vi "OVEN_Value_Indicator_Update.vi"(6 "Product Code":cluster{string, "ACTUAL  PLC COUNT":i32}[](array[cluster]), 7 "Cluster":T1={"Product List"=[], "SQL reference"=refnum, "Indicator refrence"=[], "Station Number"=[], "Shift Time stamp"=[timestamp(3597615000 s since 1904-01-01), timestamp(3597658199 s since 1904-01-01), timestamp(3597658200 s since 1904-01-01), timestamp(3597614999 s since 1904-01-01), timestamp(3597589800 s since 1904-01-01), timestamp(3597589800 s since 1904-01-01)], "Com Status Station"=[], "ALARAM INDICATOR REF"=[], "Reading"=[], "Read Parameteres"=[], "Station Name"=[], "Oven Read Parameteres"=[]} {"Shift Time stamp" format="%<%X>T"}, 8 "Machine_Number":string, 9 "Numeric":i32, 10 "Array":string[](array[string]), 11 "Cluster in":refnum<vi>) -> (3 "Boolen value of oven":bool)   [LabVIEW 2017]
uses:
  Controls/station_wise_loop_data.ctl
  <vilib>/addons/database/Connection.llb/Conn ObjectReference.ctl
  <vilib>/addons/database/NI_Database_API.lvlib
panel:
  out "400T-2 OVEN COM 2":bool
  out "Machine para Indicator":bool
  in  "Top_zone_1":dbl format="%#_13g"
  out "Read Parameteres 3":string[][](array[string])
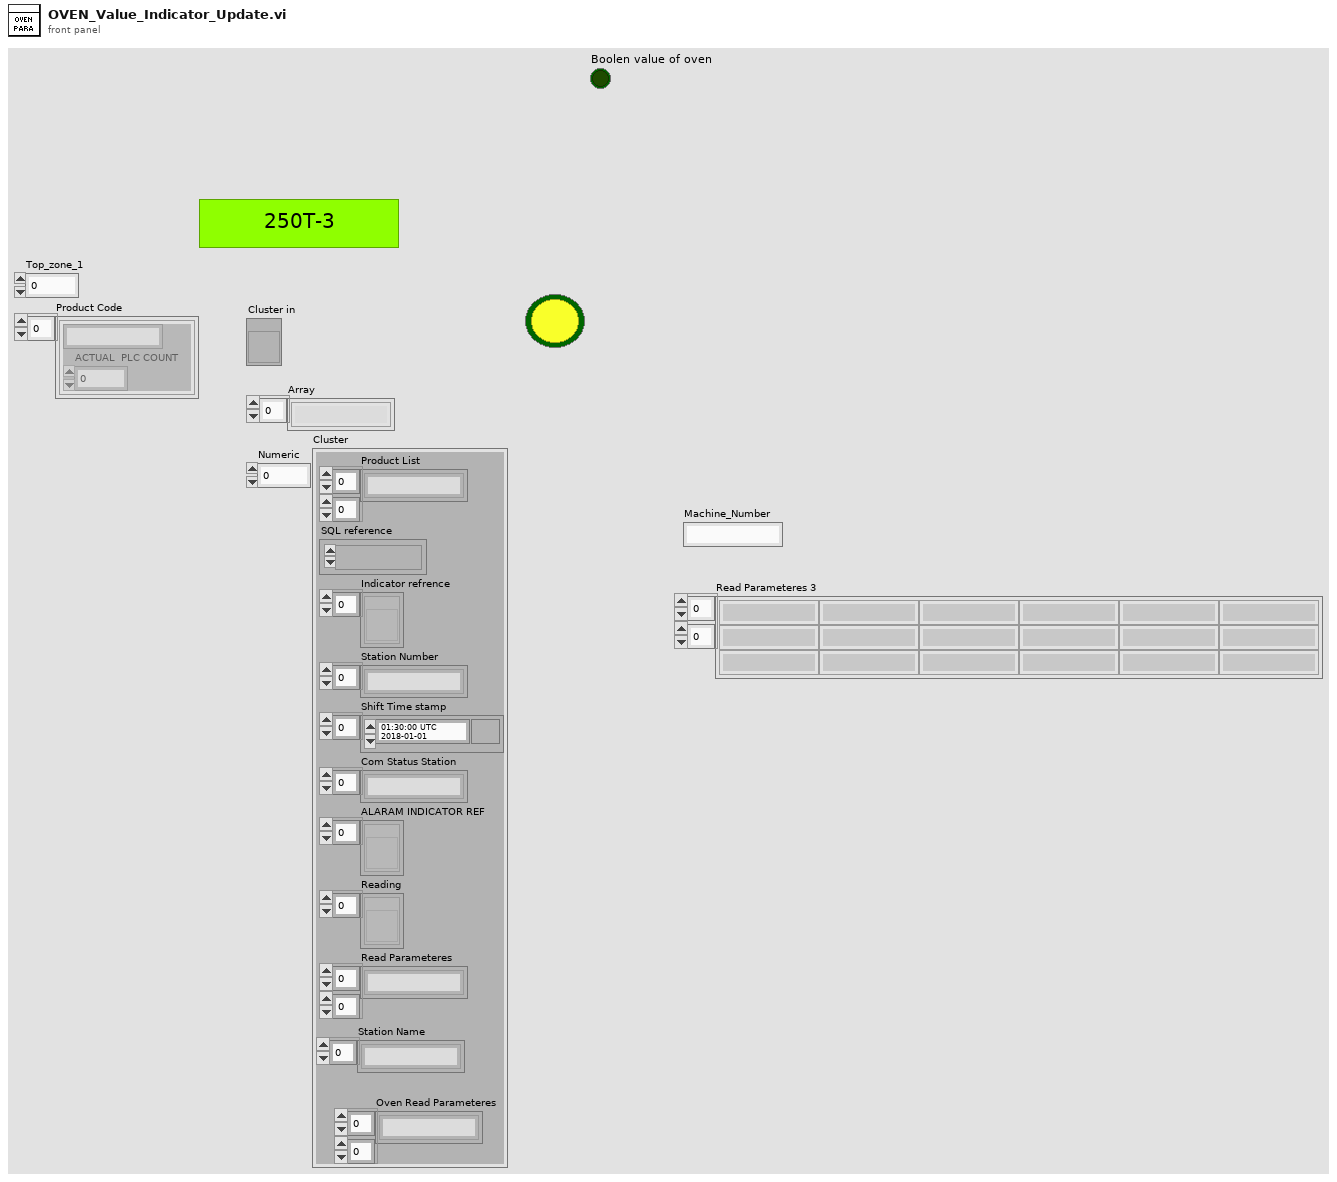
[diagram p1: front panel]
types:
  T1 = typedef "station_wise_loop_data.ctl" = cluster{"Product List":string[][], "SQL reference":T2, "Indicator refrence":refnum<vi>[], "Station Number":string[], "Shift Time stamp":timestamp[], "Com Status Station":string[], "ALARAM INDICATOR REF":refnum<vi>[], "Reading":refnum<vi>[], "Read Parameteres":string[][], "Station Name":string[], "Oven Read Parameteres":string[][]}
  T2 = typedef "NI_Database_API.lvlib/Conn ObjectReference.ctl" = refnum<k1>
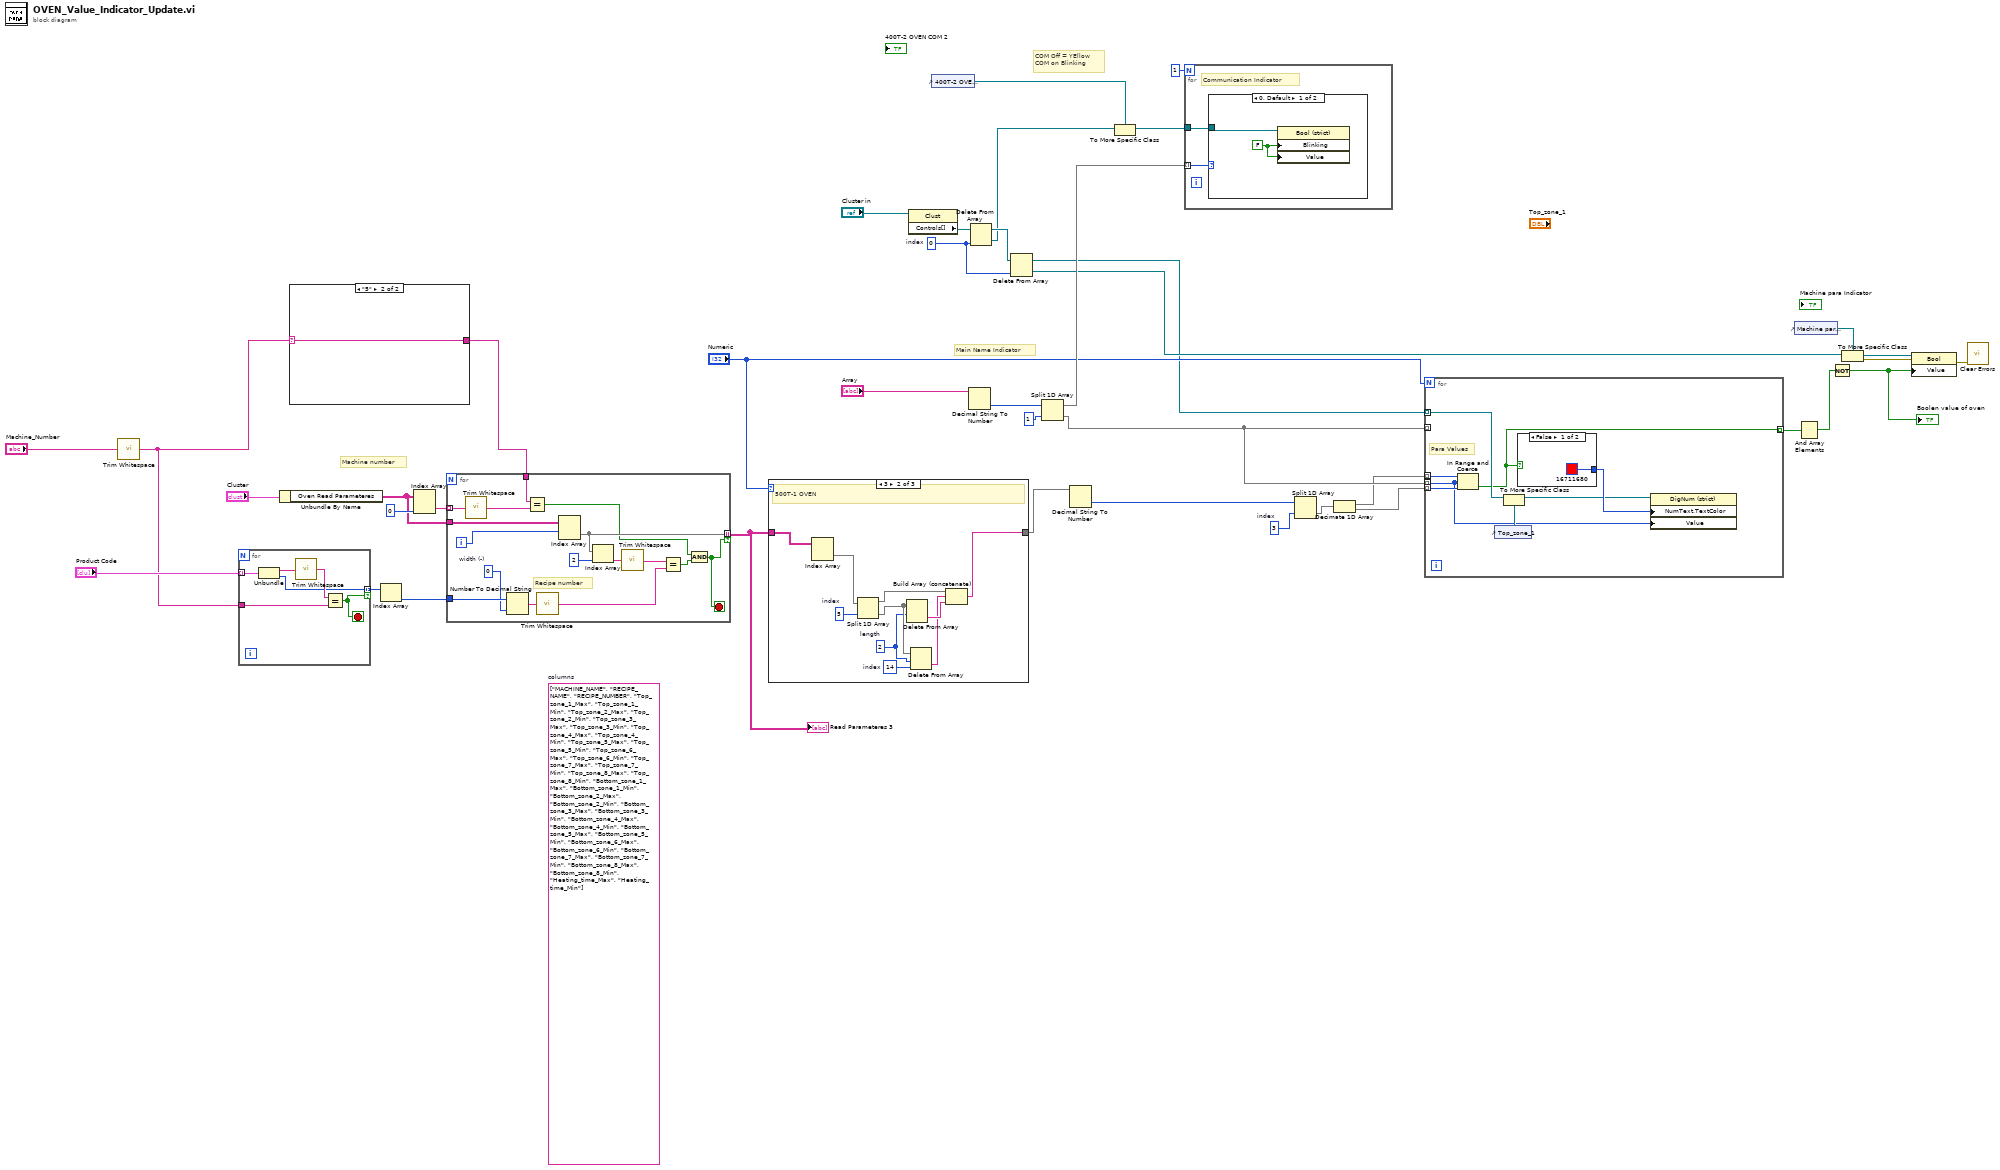
[diagram p0: block diagram]
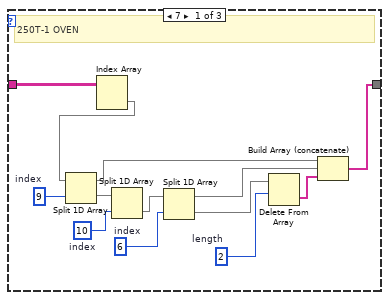
[diagram p3: hidden frame]
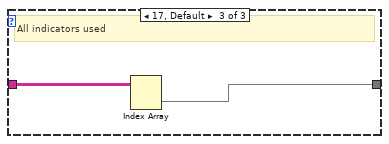
[diagram p4: hidden frame]
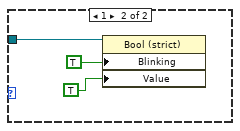
[diagram p5: hidden frame]
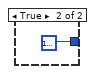
[diagram p6: hidden frame]
diagram:
  (unwired) string[] ["MACHINE_NAME", "RECIPE_NAME", "RECIPE_NUMBER", "Top_zone_1_Max", "Top_zone_1_Min", "Top_zone_2_Max", "Top_zone_2_Min", "Top_zone_3_Max", "Top_zone_3_Min", "Top_zone_4_Max", "Top_zone_4_Min", "Top_zone_5_Max", "Top_zone_5_Min", "Top_zone_6_Max", "Top_zone_6_Min", "Top_zone_7_Max", "Top_zone_7_Min", "Top_zone_8_Max", "Top_zone_8_Min", "Bottom_zone_1_Max", "Bottom_zone_1_Min", "Bottom_zone_2_Max", "Bottom_zone_2_Min", "Bottom_zone_3_Max", "Bottom_zone_3_Min", "Bottom_zone_4_Max", "Bottom_zone_4_Min", "Bottom_zone_5_Max", "Bottom_zone_5_Min", "Bottom_zone_6_Max", "Bottom_zone_6_Min", "Bottom_zone_7_Max", "Bottom_zone_7_Min", "Bottom_zone_8_Max", "Bottom_zone_8_Min", "Heating_time_Max", "Heating_time_Min"]  # columns
  w24 = 3  # index
  w32 = 0  # index
  # "Machine number"
  # "Main Name Indicator"
  # "COM Off = YEllow\nCOM on Blinking"
  n1 = call <vilib>:"Trim Whitespace.vi"("string"="Machine_Number") -> ("trimmed string"=w13:string)  [unwired: 1 in]
  n2 = for {
    tunnel: "Product Code" -> [w46] mode=indexing
    tunnel: w13 -> [w43]
    tunnel: [w42] -> w18 mode=indexing if=w41
    stop <- w41 stop-if-true
    n3 = Unbundle(w46) -> (w45:string, "ACTUAL  PLC COUNT"=w42:i32)
    n4 = call <vilib>:"Trim Whitespace.vi"("string"=w45) -> ("trimmed string"=w44:string)  [unwired: 1 in]
    n5 = Equal?(x=w44, y=w43) -> (x = y?=w41:bool)
  }
  n6 = Unbundle By Name("Cluster") -> ("Oven Read Parameteres"=w25:string[][])
  n7 = case shown="\"5\"" w13 {
    selector: w13 -> [w47 w48]
    tunnel: [w47 w48] -> w12
    frame "False", Default {
    }
    frame "5" {
    }
  }
  n8 = Index Array(array=w18) -> (element=w17:i32)  [unwired: 1 in]
  n9 = Index Array(array=w25, index (col)=0 ("disabled index (col)")) -> (element=w28:string[])  [unwired: 1 in]
  n10 = for {
    tunnel: w28 -> [w64] mode=indexing
    tunnel: w12 -> [w62]
    tunnel: w25 -> [w60]
    tunnel: [w59] -> w3 mode=indexing if=w49
    tunnel: w17 -> [w53]
    i -> [w61]
    stop <- w49 stop-if-true
    w50 = i16 0  # width (-)
    # "Recipe number"
    n11 = call <vilib>:"Trim Whitespace.vi"("string"=w64) -> ("trimmed string"=w63:string)  [unwired: 1 in]
    n12 = Number To Decimal String(number=w53, width (-)=w50) -> (decimal integer string=w52:string)
    n13 = Equal?(x=w62, y=w63) -> (x = y?=w54:bool)
    n14 = call <vilib>:"Trim Whitespace.vi"("string"=w52) -> ("trimmed string"=w51:string)  [unwired: 1 in]
    n15 = Index Array(array=w60, index (row)=w61) -> (element=w59:string[])  [unwired: 1 in]
    n16 = Index Array(array=w59, index=2) -> (element=w57:string)
    n17 = call <vilib>:"Trim Whitespace.vi"("string"=w57) -> ("trimmed string"=w56:string)  [unwired: 1 in]
    n18 = Equal?(x=w56, y=w51) -> (x = y?=w55:bool)
    n19 = And(x=w54, y=w55) -> (x .and. y?=w49:bool)
  }
  "Read Parameteres 3" <- w3
  n20 = case shown="3" "Numeric" {
    tunnel: [w68 w83 w88] -> w15
    tunnel: w3 -> [w77 w85 w89]
    frame 7 {
      w65 = 2  # length
      w67 = 6  # index
      w71 = 10  # index
      w70 = 9  # index
      # "250T-1 OVEN"
      n21 = Index Array(array=w77) -> (element=w69:string[])  [unwired: 2 in]
      n22 = Split 1D Array(array=w69, index=w70) -> (first subarray=w72:string[], second subarray=w73:string[])
      n23 = Split 1D Array(array=w73, index=w71) -> (second subarray=w66:string[])  [unwired: 1 out]
      n24 = Split 1D Array(array=w66, index=w67) -> (first subarray=w74:string[], second subarray=w76:string[])
      n25 = Delete From Array(array=w76, length=w65) -> (deleted portion=w75:string[])  [unwired: 1 in, 1 out]
      n26 = Build Array (concatenate)(w72, w74, w75) -> (w68:string[])
    }
    frame 3 {
      w80 = 14  # index
      w79 = 2  # length
      w87 = 5  # index
      # "500T-1 OVEN"
      n27 = Index Array(array=w85) -> (element=w84:string[])  [unwired: 2 in]
      n28 = Split 1D Array(array=w84, index=w87) -> (first subarray=w82:string[], second subarray=w81:string[])
      n29 = Delete From Array(array=w81, length=w79) -> (deleted portion=w86:string[])  [unwired: 1 in, 1 out]
      n30 = Delete From Array(array=w81, length=w79, index=w80) -> (deleted portion=w78:string[])  [unwired: 1 out]
      n31 = Build Array (concatenate)(w82, w78, w86) -> (w83:string[])
    }
    frame 17, Default {
      # "All indicators used"
      n32 = Index Array(array=w89) -> (element=w88:string[])  [unwired: 2 in]
    }
  }
  n33 = property on="Property Node" class="Clust"(reference="Cluster in") -> ("Controls[]"=w38:refnum<vi>[])  [unwired: 1 in, 2 out]
  n34 = control-ref of="400T-2 OVEN COM 2"() -> (w2:refnum<vi>)
  n35 = Decimal String To Number(string="Array") -> (number=w36:i32[])  [unwired: 2 in, 1 out]
  n36 = Delete From Array(array=w38, index=w32) -> (deleted portion=w31:refnum<vi>, array with subset deleted=w33:refnum<vi>[])  [unwired: 1 in]
  n37 = Delete From Array(array=w33, index=w32) -> (deleted portion=w5:refnum<vi>, array with subset deleted=w1:refnum<vi>[])  [unwired: 1 in]
  n38 = Split 1D Array(array=w36, index=1) -> (first subarray=w35:i32[], second subarray=w29:i32[])
  n39 = Decimal String To Number(string=w15) -> (number=w23:i32[])  [unwired: 2 in, 1 out]
  n40 = To More Specific Class(target class=w2, reference=w31) -> (specific class reference=w30:refnum<vi>)  [unwired: 1 in, 1 out]
  n41 = for {
    N: 1 -> [_]
    tunnel: w30 -> [w91]
    tunnel: w35 -> [w90] mode=indexing
    # "Communication Indicator"
    n42 = case shown="0, Default" w90 {
      tunnel: w91 -> [w93 w96]
      frame 0, Default {
        w92 = FALSE
        n43 = property on="Property Node" class="Bool (strict)"(reference=w93, "Blinking"=w92, "Value"=w92) -> ()  [unwired: 1 in, 2 out]
      }
      frame 1 {
        n44 = property on="Property Node" class="Bool (strict)"(reference=w96, "Blinking"=TRUE, "Value"=TRUE) -> ()  [unwired: 1 in, 2 out]
      }
    }
  }
  n45 = Split 1D Array(array=w23, index=w24) -> (second subarray=w20:i32[])  [unwired: 1 out]
  n46 = Decimate 1D Array(w20) -> (w22:i32[], w21:i32[])
  n47 = for {
    N: "Numeric" -> [_]
    tunnel: w29 -> [_] mode=indexing
    tunnel: w1 -> [w100] mode=indexing
    tunnel: w29 -> [w98] mode=indexing
    tunnel: w22 -> [w104] mode=indexing
    tunnel: w21 -> [w103] mode=indexing
    tunnel: [w97] -> w6 mode=indexing
    # "Para Values"
    n48 = In Range and Coerce(upper limit=w104, x=w98, lower limit=w103) -> (In Range?=w97:bool)  [unwired: 1 out]
    n49 = control-ref of="Top_zone_1"() -> (w101:refnum<vi>)
    n50 = To More Specific Class(target class=w101, reference=w100) -> (specific class reference=w99:refnum<vi>)  [unwired: 1 in, 1 out]
    n51 = case shown="False" w97 {
      tunnel: [u32 16711680 ("Numeric Text.Text Colors:BG Color 2") u32 16777222 ("Numeric Text.Text Colors:BG Color 2")] -> w102
      frame False {
      }
      frame True {
      }
    }
    n52 = property on="Property Node" class="DigNum (strict)"(reference=w99, "NumText.TextColor"=w102, "Value"=w98) -> ()  [unwired: 1 in, 2 out]
  }
  n53 = control-ref of="Machine para Indicator"() -> (w10:refnum<vi>)
  n54 = And Array Elements(Boolean array=w6) -> (logical AND=w7:bool)
  n55 = Not(x=w7) -> (.not. x?=w8:bool)
  "Boolen value of oven" <- w8
  n56 = To More Specific Class(target class=w10, reference=w5) -> (specific class reference=w9:refnum<vi>, error out=w11:errorcluster)  [unwired: 1 in]
  n57 = property on="Property Node" class="Bool"(reference=w9, error in=w11, "Value"=w8) -> (error out=w4:errorcluster)  [unwired: 1 out]
  n58 = call <vilib>:"Clear Errors.vi"("error in (no error)"=w4) -> ()  [unwired: 5 in, 2 out]
